vi "Generate SPI Write Data Frame.vi"(11 "Data":u16 format="%.0x") -> (3 "SPI Write Data Frame":bool[](array[boolean]))   [LabVIEW 2023, in "SPI.lvlib"]
uses:
  SPI.lvlib
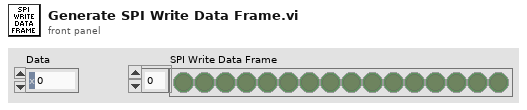
[diagram p1: front panel]
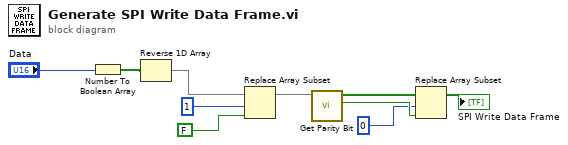
[diagram p0: block diagram]
diagram:
  n1 = Number To Boolean Array(number="Data") -> (Boolean array=w9:bool[])
  n2 = Reverse 1D Array(array=w9) -> (reversed array=w8:bool[])
  n3 = Replace Array Subset(array=w8, new element=FALSE ("new element/subarray"), index=1) -> (w6:bool[])
  n4 = call "Get Parity Bit.vi"("Array in"=w6) -> ("Parity Bit"=w4:bool, "Array out"=w5:bool[])  [unwired: 9 in]
  n5 = Replace Array Subset(array=w5, new element=w4, index=0) -> (→"SPI Write Data Frame":bool[])
